vi "Stop Acquire.vi"(8 "error in (no error)":errorcluster, 11 "Measure Object in":refnum<class "Measure Object.lvclass">) -> (0 "error out":errorcluster, 3 "Measure Object out":refnum<class "Measure Object.lvclass">)   [LabVIEW 2016, in "Measure Object.lvclass"]
uses:
  Measure Object.lvclass
  Measure Object.lvclass/Measure Object.ctl
  Write Active.vi
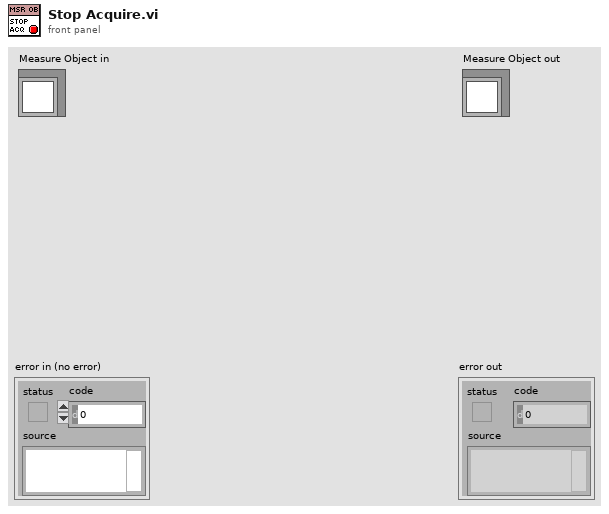
[diagram p1: front panel]
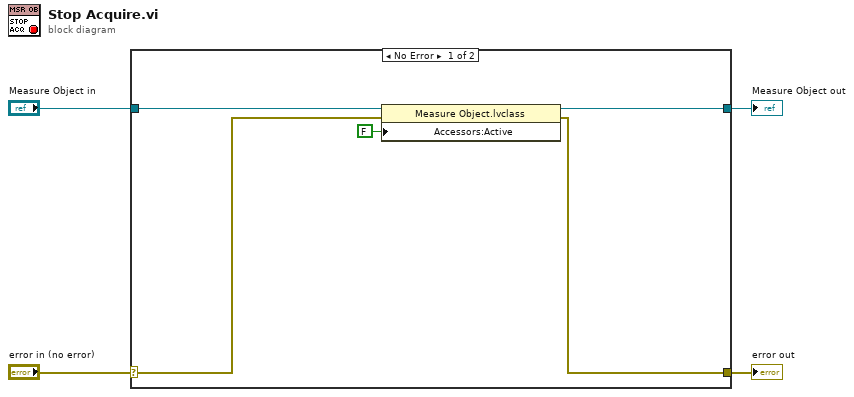
[diagram p0: block diagram]
diagram:
  n1 = case shown="No Error" "error in (no error)" {
    selector: "error in (no error)" -> [w6 w11]
    tunnel: [w5 w11] -> w3
    tunnel: [w8 w10] -> w1
    tunnel: "Measure Object in" -> [w9 w10]
    frame No Error {
      n2 = property class="Measure Object.lvclass"(reference=w9, error in=w6, "Accessors:Active"=FALSE ("Active")) -> (reference out=w8:refnum<class "Measure Object.lvclass">, error out=w5:errorcluster)
    }
    frame Error {
    }
  }
  "error out" <- w3
  "Measure Object out" <- w1
